vi "_CSTK_Button_Icon_Config_UpdateConfiguration.vi"(8 "error in (no error)":errorcluster caption="错误输入（无错误）", 9 "Update Index":i32, 10 "Configuration in":T1, 11 "State 输入":T3 caption="State in") -> (0 "error out":errorcluster, 2 "Configuration out":T1={"背景颜色"=0, "LOGO"={"显示LOGO"=FALSE, "水平偏移"=0, "LOGO路径"=path "", "LOGO图片"=bytes[0]}, "布尔文本"={"显示文本"=FALSE, "水平偏移"=0, "布尔文本"="", "文本颜色"=0, "字体样式"={"Font Name"="", "Size"=17, "Strikeout?"=FALSE, "Italic?"=FALSE, "Underline?"=FALSE, "Outline?"=FALSE, "Shadow?"=FALSE, "Bold?"=FALSE}}, "边框"={"颜色"=0, "线条宽度"=0, "圆角半径"=0, "线条样式"=enum."Solid"}}, 3 "State 输出":T3 caption="State out")   [LabVIEW 2015, in "CSTK_Button_Icon.xctl"]
uses:
  CSTK_Button_Icon.xctl
  TypeDefinitions/CSTK_Button_Icon_Properties_Configure.ctl
  TypeDefinitions/_CSTK_Button_Icon_TextProperties_FontStyle.ctl
  CSTK_Button_Icon_Status.ctl
  TypeDefinitions/_CSTK_Button_Icon_ButtonSize.ctl
  <vilib>/Utility/miscctls.llb/LVBoundsTypeDef.ctl
  TypeDefinitions/_CSTK_Button_Icon_LogoImage.ctl
  <vilib>/picture/picture.llb/imagedata.ctl
  TypeDefinitions/_CSTK_Button_Icon_LogoProperties.ctl
  TypeDefinitions/_CSTK_Button_Icon_LogoProperties_Data.ctl
  TypeDefinitions/_CSTK_Button_Icon_TextString.ctl
  TypeDefinitions/_CSTK_Button_Icon_TextProperties.ctl
  TypeDefinitions/_CSTK_Button_Icon_TextProperties_Data.ctl
  TypeDefinitions/_CSTK_Button_Icon_BGColor.ctl
  TypeDefinitions/_CSTK_Button_Icon_BorderColor.ctl
  TypeDefinitions/_CSTK_Button_Icon_BorderProperties.ctl
  TypeDefinitions/_CSTK_Button_Icon_BorderProperties_Data.ctl
  TypeDefinitions/_CSTK_Button_Icon_CurrentBGImage.ctl
  TypeDefinitions/_CSTK_Button_Icon_DrawAreaSize.ctl
  TypeDefinitions/_CSTK_Button_Icon_TextStartOffset.ctl
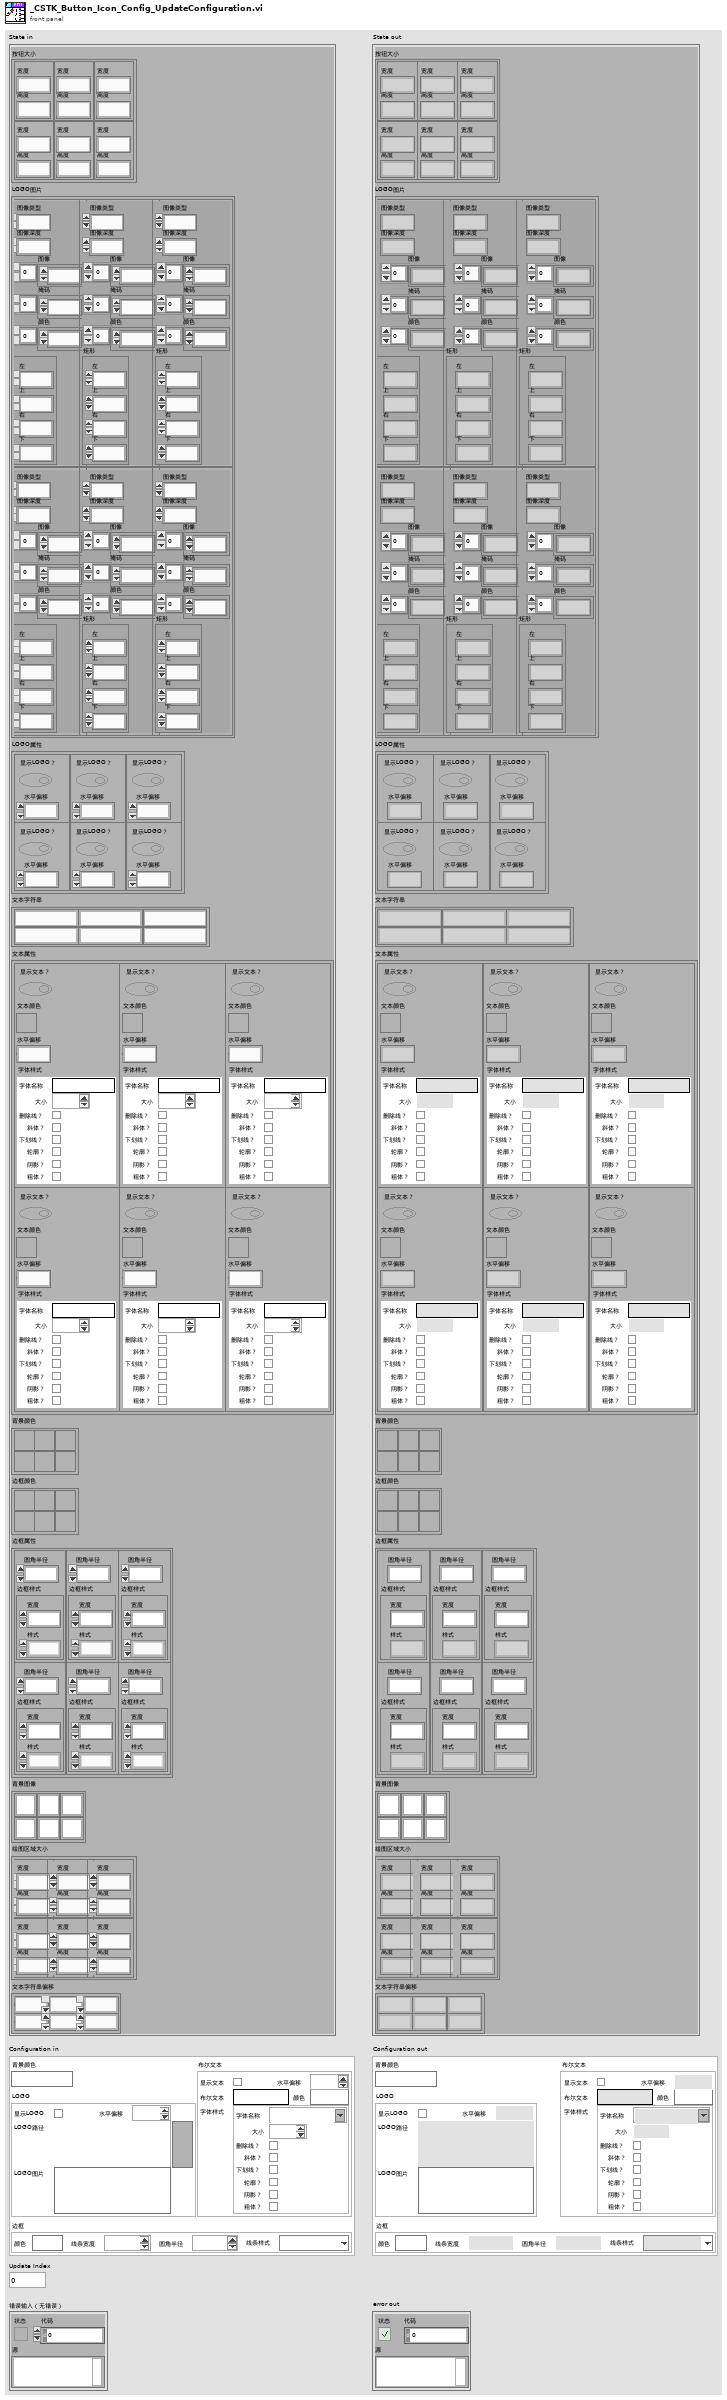
[diagram p1: front panel]
types:
  T1 = typedef "CSTK_Button_Icon.xctl/CSTK_Button_Icon_Properties_Configure.ctl" = cluster{"背景颜色":u32, "LOGO":cluster{"显示LOGO":bool, "水平偏移":i16, "LOGO路径":path, "LOGO图片":picture}, "布尔文本":cluster{"显示文本":bool, "水平偏移":i16, "布尔文本":string, "文本颜色":u32, "字体样式":T2}, "边框":cluster{"颜色":u32, "线条宽度":u16, "圆角半径":i16, "线条样式":enum32{"Solid", "Dash", "Dot", "DashDot", "DashDotDot"}}}
  T2 = typedef "CSTK_Button_Icon.xctl/_CSTK_Button_Icon_TextProperties_FontStyle.ctl" = cluster{"Font Name":string, "Size":i16, "Strikeout?":bool, "Italic?":bool, "Underline?":bool, "Outline?":bool, "Shadow?":bool, "Bold?":bool}
  T3 = typedef "CSTK_Button_Icon.xctl/CSTK_Button_Icon_Status.ctl" = cluster{"ButtonSize":T4, "Logo Image":T6, "Logo Properties":T8, "Text String":T10, "Text Properties":T11, "BG Color":T13, "Border Color":T14, "Border Properties":T15, "Current BG Image":T17, "DrawAreaSize":T18, "Text String Offset":T19}
  T4 = typedef "CSTK_Button_Icon.xctl/_CSTK_Button_Icon_ButtonSize.ctl" = cluster{"False":T5, "True":T5, "True to False":T5, "False to True":T5, "Hover in False":T5, "Hover in True":T5}
  T5 = typedef "LVBoundsTypeDef.ctl" = cluster{"Width":u32, "Height":u32}
  T6 = typedef "CSTK_Button_Icon.xctl/_CSTK_Button_Icon_LogoImage.ctl" = cluster{"False":T7, "True":T7, "True to False":T7, "False to True":T7, "Hover in False":T7, "Hover in True":T7}
  T7 = typedef "imagedata.ctl" = cluster{"image type":i32, "image depth":i32, "image":u8[], "mask":u8[], "colors":u32[], "Rectangle":cluster{"left":i16, "top":i16, "right":i16, "bottom":i16}}
  T8 = typedef "CSTK_Button_Icon.xctl/_CSTK_Button_Icon_LogoProperties.ctl" = cluster{"False":T9, "True":T9, "True to False":T9, "False to True":T9, "Hover in False":T9, "Hover in True":T9}
  T9 = typedef "CSTK_Button_Icon.xctl/_CSTK_Button_Icon_LogoProperties_Data.ctl" = cluster{"Display Logo?":bool, "Horizontal Offset":i16}
  T10 = typedef "CSTK_Button_Icon.xctl/_CSTK_Button_Icon_TextString.ctl" = cluster{"False":string, "True":string, "True to False":string, "False to True":string, "Hover in False":string, "Hover in True":string}
  T11 = typedef "CSTK_Button_Icon.xctl/_CSTK_Button_Icon_TextProperties.ctl" = cluster{"False":T12, "True":T12, "True to False":T12, "False to True":T12, "Hover in False":T12, "Hover in True":T12}
  T12 = typedef "CSTK_Button_Icon.xctl/_CSTK_Button_Icon_TextProperties_Data.ctl" = cluster{"Display Text?":bool, "Text Color":u32, "Horizontal Offset":i16, "Font Style":T2}
  T13 = typedef "CSTK_Button_Icon.xctl/_CSTK_Button_Icon_BGColor.ctl" = cluster{"False":u32, "True":u32, "True to False":u32, "False to True":u32, "Hover in False":u32, "Hover in True":u32}
  T14 = typedef "CSTK_Button_Icon.xctl/_CSTK_Button_Icon_BorderColor.ctl" = cluster{"False":u32, "True":u32, "True to False":u32, "False to True":u32, "Hover in False":u32, "Hover in True":u32}
  T15 = typedef "CSTK_Button_Icon.xctl/_CSTK_Button_Icon_BorderProperties.ctl" = cluster{"False":T16, "True":T16, "True to False":T16, "False to True":T16, "Hover in False":T16, "Hover in True":T16}
  T16 = typedef "CSTK_Button_Icon.xctl/_CSTK_Button_Icon_BorderProperties_Data.ctl" = cluster{"Radius":i16, "Border Style":cluster{"Width":u16, "Style":enum32{"Solid", "Dash", "Dot", "DashDot", "DashDotDot"}}}
  T17 = typedef "CSTK_Button_Icon.xctl/_CSTK_Button_Icon_CurrentBGImage.ctl" = cluster{"False":picture, "True":picture, "True to False":picture, "False to True":picture, "Hover in False":picture, "Hover in True":picture}
  T18 = typedef "CSTK_Button_Icon.xctl/_CSTK_Button_Icon_DrawAreaSize.ctl" = cluster{"False":T5, "True":T5, "True to False":T5, "False to True":T5, "Hover in False":T5, "Hover in True":T5}
  T19 = typedef "CSTK_Button_Icon.xctl/_CSTK_Button_Icon_TextStartOffset.ctl" = cluster{"False":i32, "True":i32, "True to False":i32, "False to True":i32, "Hover in False":i32, "Hover in True":i32}
  T20 = enum32{"Solid", "Dash", "Dot", "DashDot", "DashDotDot"}
  T21 = cluster{"Logo Image[0]":T7, "Logo Image[1]":T7, "Logo Image[2]":T7, "Logo Image[3]":T7, "Logo Image[4]":T7, "Logo Image[5]":T7}
  T22 = cluster{"Logo Properties[0]":T9, "Logo Properties[1]":T9, "Logo Properties[2]":T9, "Logo Properties[3]":T9, "Logo Properties[4]":T9, "Logo Properties[5]":T9}
  T23 = cluster{"Text String[0]":string, "Text String[1]":string, "Text String[2]":string, "Text String[3]":string, "Text String[4]":string, "Text String[5]":string}
  T24 = cluster{"Text Properties[0]":T12, "Text Properties[1]":T12, "Text Properties[2]":T12, "Text Properties[3]":T12, "Text Properties[4]":T12, "Text Properties[5]":T12}
  T25 = cluster{"BG Color[0]":u32, "BG Color[1]":u32, "BG Color[2]":u32, "BG Color[3]":u32, "BG Color[4]":u32, "BG Color[5]":u32}
  T26 = cluster{"Border Color[0]":u32, "Border Color[1]":u32, "Border Color[2]":u32, "Border Color[3]":u32, "Border Color[4]":u32, "Border Color[5]":u32}
  T27 = cluster{"Border Properties[0]":T16, "Border Properties[1]":T16, "Border Properties[2]":T16, "Border Properties[3]":T16, "Border Properties[4]":T16, "Border Properties[5]":T16}
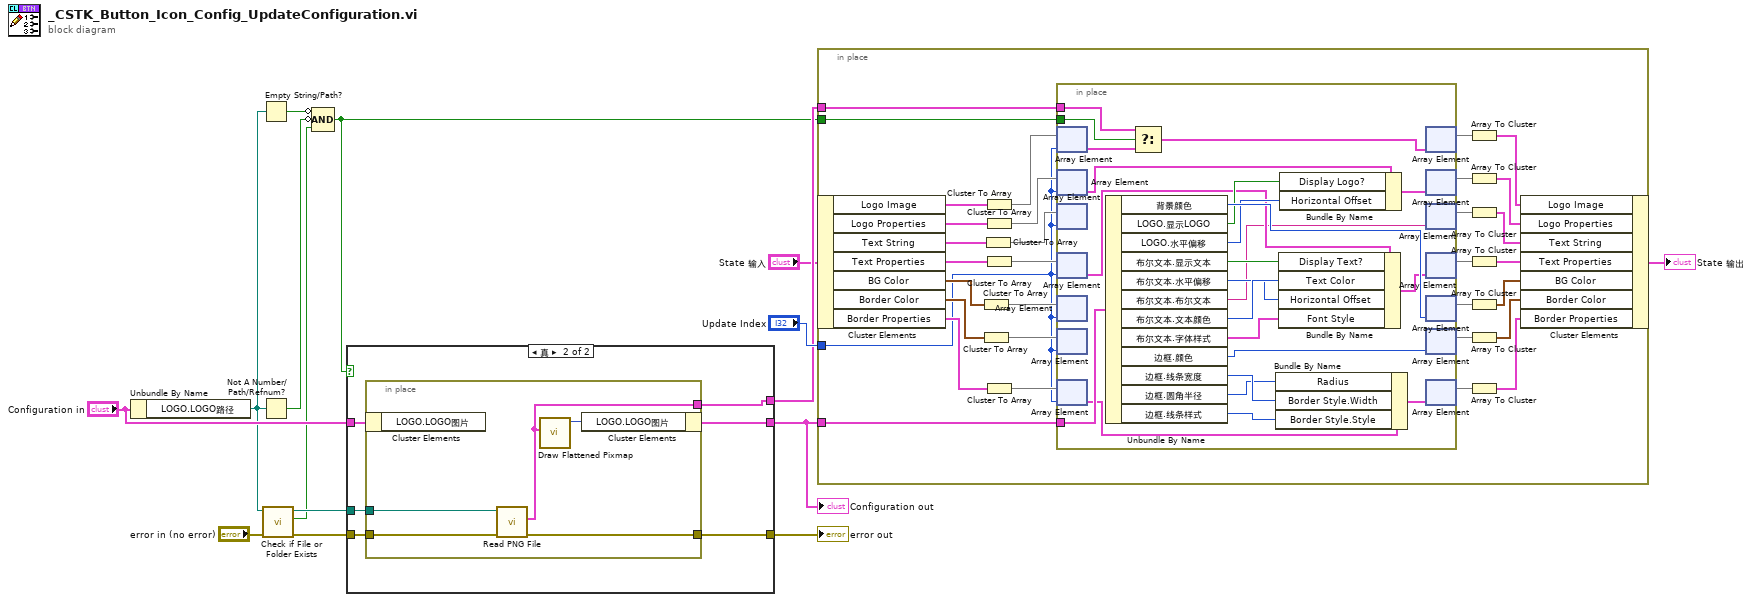
[diagram p0: block diagram]
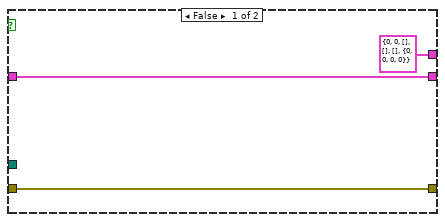
[diagram p2: hidden frame]
diagram:
  n1 = Unbundle By Name("Configuration in") -> ("LOGO.LOGO路径"=w3:path)
  n2 = Empty String/Path?(string/path=w3) -> (empty?=w4:bool)
  n3 = Not A Number/Path/Refnum?(number/path/refnum=w3) -> (NaN/Path/Refnum?=w5:bool)
  n4 = call <vilib>:"Check if File or Folder Exists.vi"("error in (no error)"="error in (no error)", "path"=w3) -> ("error out"=w10:errorcluster, "file or folder exists?"=w2:bool, "dup path"=w13:path)  [unwired: 7 in]
  n5 = Compound Arithmetic op=AND ("复合运算")(invert w4, invert w5, w2) -> (w1:bool)
  n6 = case shown="真" w1 {
    tunnel: w13 -> [_ w22]
    tunnel: "Configuration in" -> [w18 w24]
    tunnel: [w18 w23] -> w11
    tunnel: w10 -> [w17 w21]
    tunnel: [w17 w20] -> w8
    tunnel: [T7 {"image type"=0, "image depth"=0, "image"=[], "mask"=[], "colors"=[], "Rectangle"={"left"=0, "top"=0, "right"=0, "bottom"=0}} ("image data") w19] -> w7
    frame False {
    }
    frame True {
      n7 = in-place {
        in-place-border: w22 -> [w29]
        in-place-border: w21 -> [w28]
        in-place-border: [w27] -> w20
        in-place-border: [w25] -> w19
        n8 = in-place-cluster #1(w24) -> ()  [unwired: 1 out]
        n9 = call <vilib>:"Read PNG File.vi"("error in (no error)"=w28, "path to PNG file"=w29) -> ("error out"=w27:errorcluster, "image data"=w25:T7)  [unwired: 7 in, 1 out]
        n10 = call <vilib>:"Draw Flattened Pixmap.vi"("image data"=w25) -> ("new picture"=w26:picture)  [unwired: 8 in]
        n11 = in-place-cluster #1("LOGO.LOGO图片"=w26) -> (w23:T1)
      }
    }
  }
  "error out" <- w8
  "Configuration out" <- w11
  n12 = in-place {
    in-place-border: "Update Index" -> [w33]
    in-place-border: w11 -> [w32]
    in-place-border: w1 -> [w31]
    in-place-border: w7 -> [w30]
    n13 = in-place-cluster #2("State 输入") -> ("Logo Image"=w54:T6, "Logo Properties"=w53:T8, "Text String"=w52:T10, "Text Properties"=w51:T11, "BG Color"=w50:T13, "Border Color"=w49:T14, "Border Properties"=w48:T15)
    n14 = Cluster To Array(cluster=w50) -> (array=w57:u32[])
    n15 = Cluster To Array(cluster=w49) -> (array=w56:u32[])
    n16 = Cluster To Array(cluster=w52) -> (array=w59:string[])
    n17 = Cluster To Array(cluster=w54) -> (array=w61:T7[])
    n18 = Cluster To Array(cluster=w53) -> (array=w60:T9[])
    n19 = Cluster To Array(cluster=w51) -> (array=w58:T12[])
    n20 = Cluster To Array(cluster=w48) -> (array=w55:T16[])
    n21 = in-place {
      in-place-border: w32 -> [w84]
      in-place-border: w31 -> [w82]
      in-place-border: w30 -> [w81]
      n22 = in-place-array #3(w61, w33) -> (w79:T7)
      n23 = in-place-array #4(w60, w33) -> (w78:T9)
      n24 = in-place-array #5(w59, w33) -> ()  [unwired: 1 out]
      n25 = in-place-array #6(w58, w33) -> (w74:T12)
      n26 = in-place-array #7(w57, w33) -> ()  [unwired: 1 out]
      n27 = in-place-array #8(w56, w33) -> ()  [unwired: 1 out]
      n28 = in-place-array #9(w55, w33) -> (w66:T16)
      n29 = Unbundle By Name(w84) -> ("背景颜色"=w83:u32, "LOGO.显示LOGO"=w77:bool, "LOGO.水平偏移"=w76:i16, "布尔文本.显示文本"=w73:bool, "布尔文本.水平偏移"=w70:i16, "布尔文本.布尔文本"=w68:string, "布尔文本.文本颜色"=w71:u32, "布尔文本.字体样式"=w69:T2, "边框.颜色"=w67:u32, "边框.线条宽度"=w65:u16, "边框.圆角半径"=w64:i16, "边框.线条样式"=w63:T20)
      n30 = Select(t=w81, s=w82, f=w79) -> (s? t:f=w80:T7)
      n31 = Bundle By Name(cluster=w66, "Radius"=w64, "Border Style.Width"=w65, "Border Style.Style"=w63) -> (w62:T16)
      n32 = Bundle By Name(cluster=w74, "Display Text?"=w73, "Text Color"=w71, "Horizontal Offset"=w70, "Font Style"=w69) -> (w72:T12)
      n33 = Bundle By Name(cluster=w78, "Display Logo?"=w77, "Horizontal Offset"=w76) -> (w75:T9)
      n34 = in-place-array #3(w80) -> (w47:T7[])  [unwired: 1 out]
      n35 = in-place-array #4(w75) -> (w45:T9[])  [unwired: 1 out]
      n36 = in-place-array #5(w68) -> (w44:string[])  [unwired: 1 out]
      n37 = in-place-array #6(w72) -> (w43:T12[])  [unwired: 1 out]
      n38 = in-place-array #7(w83) -> (w42:u32[])  [unwired: 1 out]
      n39 = in-place-array #8(w67) -> (w41:u32[])  [unwired: 1 out]
      n40 = in-place-array #9(w62) -> (w40:T16[])  [unwired: 1 out]
    }
    n41 = Array To Cluster(array=w47) -> (cluster=w46:T21)
    n42 = Array To Cluster(array=w45) -> (cluster=w39:T22)
    n43 = Array To Cluster(array=w44) -> (cluster=w38:T23)
    n44 = Array To Cluster(array=w43) -> (cluster=w37:T24)
    n45 = Array To Cluster(array=w42) -> (cluster=w36:T25)
    n46 = Array To Cluster(array=w41) -> (cluster=w35:T26)
    n47 = Array To Cluster(array=w40) -> (cluster=w34:T27)
    n48 = in-place-cluster #2("Logo Image"=w46, "Logo Properties"=w39, "Text String"=w38, "Text Properties"=w37, "BG Color"=w36, "Border Color"=w35, "Border Properties"=w34) -> (→"State 输出":T3)
  }
